vi "WPI_DigitalOutputGetPWM.vi"(8 "error in (no error)":errorcluster, 11 "DigitalOutputDevRef":T1={"DIO Channel"=enum."DIO 1", "DevStatus"={"status"=FALSE, "code"=0, "source"=""}}) -> (0 "error out":errorcluster, 2 "PWM Duty Cycle":sgl, 3 "DigitalOutputDevRef":T1={"DIO Channel"=enum."DIO 1", "DevStatus"={"status"=FALSE, "code"=0, "source"=""}})   [LabVIEW 2017]
doc: "Generates a PWM signal on a Digital Output channel.\n\nThe resolution of the duty cycle is 8-bit for low frequencies (1kHz or less) but is reduced the higher the frequency of the PWM signal is.\n\nThis software is licensed. Open the labview\\readme\\WPI Robotics Library Open Source License.txt file for more information."
uses:
  <vilib>/Rock Robotics/WPI/DigitalOutput/WPI_DigitalOutputDevRef.ctl
  <vilib>/Rock Robotics/SystemInterfaces/DIO/FPGA_DIOChannel.ctl
  <vilib>/Rock Robotics/WPI/DigitalModule/WPI_DigitalModuleDIOCacheOp.ctl
  <vilib>/Rock Robotics/SystemInterfaces/System/FPGA_SystemGet.vi
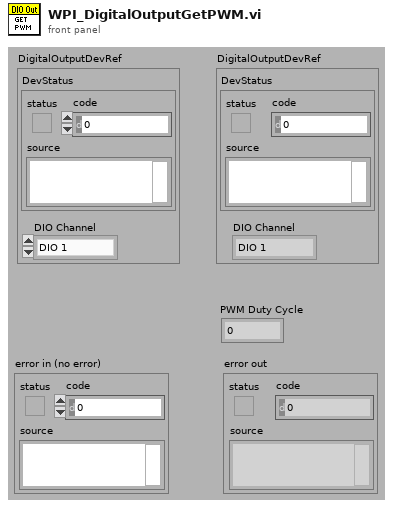
[diagram p1: front panel]
types:
  T1 = typedef "WPI_DigitalOutputDevRef.ctl" = cluster{"DIO Channel":T2, "DevStatus":errorcluster}
  T2 = typedef "FPGA_DIOChannel.ctl" = enum8{"DIO 0", "DIO 1", "DIO 2", "DIO 3", "DIO 4", "DIO 5", "DIO 6", "DIO 7", "DIO 8", "DIO 9", "DIO MXP 0", "DIO MXP 1", "DIO MXP 2", "DIO MXP 3", "DIO MXP 4", "DIO MXP 5", "DIO MXP 6", "DIO MXP 7", "DIO MXP 8", "DIO MXP 9", "DIO MXP 10", "DIO MXP 11", "DIO MXP 12", "DIO MXP 13", "DIO MXP 14", "DIO MXP 15", "SPI Port CS1", "SPI Port CS2", "SPI Port CS3", "SPI Port MISO", "SPI Port MOSI", "Invalid"}
  T3 = typedef "WPI_DigitalModuleDIOCacheOp.ctl" = enum16{"Acquire", "Release", "Status"}
  T4 = typedef "WPI_DigitalOutputPWMRef.ctl" = enum16{"DO PWM 0", "DO PWM 1", "DO PWM 2", "DO PWM 3", "DO PWM 4", "DO PWM 5", "Invalid"}
  T5 = typedef "FPGA_DIODevRef.ctl" = cluster{"DevStatus":errorcluster}
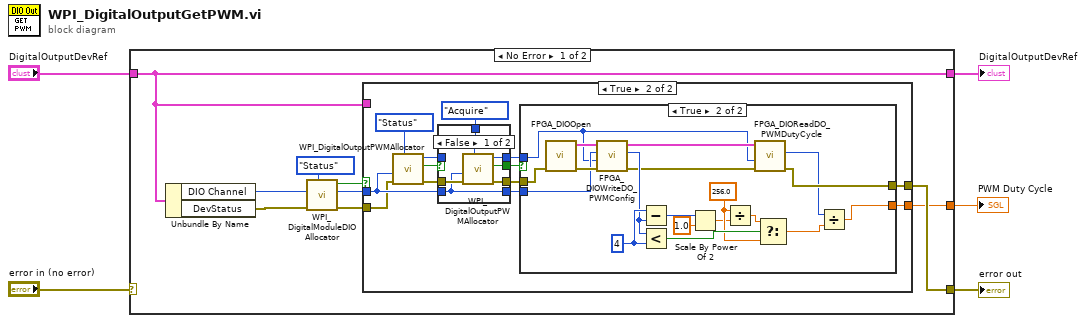
[diagram p0: block diagram]
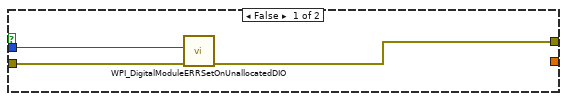
[diagram p2: hidden frame]
diagram:
  n1 = case shown="No Error" "error in (no error)" {
    selector: "error in (no error)" -> [_ w62]
    tunnel: "DigitalOutputDevRef" -> [w7 w61]
    tunnel: [w7 w61] -> w4
    tunnel: [w8 w62] -> w2
    tunnel: [w6 _] -> w1
    frame No Error {
      n2 = Unbundle By Name(w7) -> ("DIO Channel"=w13:T2, "DevStatus"=w12:errorcluster)
      n3 = call <vilib>:"WPI_DigitalModuleDIOAllocator.vi"("AllocatedDIOMutex"=WPI_DigitalModuleDIOCacheOp."Status", "error in (no error)"=w12, "DIOChannel"=w13) -> ("error out"=w9:errorcluster, "Allocated DIOChannel"=w11:T2, "AllocatedDIO"=w10:bool)  [unwired: 1 in, 5 out]
      n4 = case shown="True" w10 {
        tunnel: [w16 w19] -> w8
        tunnel: w11 -> [w15 w26]
        tunnel: w7 -> [_ _]
        tunnel: w9 -> [w17 w25]
        tunnel: [_ w18] -> w6
        frame False {
          n5 = call <vilib>:"WPI_DigitalModuleERRSetOnUnallocatedDIO.vi"("error in (no error)"=w17, "DIOChannel"=w15) -> ("error out"=w16:errorcluster)  [unwired: 9 in]
        }
        frame True {
          n6 = call <vilib>:"WPI_DigitalOutputPWMAllocator.vi"("Operation"=WPI_DigitalModuleDIOCacheOp."Status", "error in (no error)"=w25, "DIO Channel"=w26) -> ("error out"=w24:errorcluster, "Allocated"=w29:bool, "PWM Allocated"=w28:T4)  [unwired: 2 in, 4 out]
          n7 = case shown="False" w29 {
            selector: w29 -> [_ w58]
            tunnel: w28 -> [_ w60]
            tunnel: [w56 w60] -> w22
            tunnel: WPI_DigitalModuleDIOCacheOp."Acquire" ("Operation") -> [w55 _]
            tunnel: w26 -> [w51 w57]
            tunnel: w24 -> [w54 w59]
            tunnel: [w53 w59] -> w20
            tunnel: [w52 w58] -> w23
            tunnel: [w51 w57] -> w21
            frame False {
              n8 = call <vilib>:"WPI_DigitalOutputPWMAllocator.vi"("Operation"=w55, "error in (no error)"=w54, "DIO Channel"=w51) -> ("error out"=w53:errorcluster, "Allocated"=w52:bool, "PWM Allocated"=w56:T4)  [unwired: 2 in, 4 out]
            }
            frame True {
            }
          }
          n9 = case shown="True" w23 {
            tunnel: w22 -> [_ w36]
            tunnel: w21 -> [_ w47]
            tunnel: w20 -> [w31 w49]
            tunnel: [w31 w33] -> w19
            tunnel: [_ w34] -> w18
            frame False {
            }
            frame True {
              w45 = u8 4 ("y")
              w43 = 256.0 ("y")
              n10 = call <vilib>:"FPGA_DIOOpen.vi"("error in (no error)"=w49) -> ("error out"=w48:errorcluster, "DIODeviceRef"=w50:T5)  [unwired: 1 in, 8 out]
              n11 = call <vilib>:"FPGA_DIOWriteDO_PWMConfig.vi"("error in (no error)"=w48, "DO_PWM Index"=w36, "DO_PWMOutputSelect"=w47, "DIODeviceRef"=w50) -> ("error out"=w37:errorcluster, "DO_PWMPeriodPower Out"=w44:u16, "DIODeviceRef"=w38:T5)  [unwired: 1 in, 4 out]
              n12 = Subtract(x=w45, y=w44) -> (x-y=w40:u16)
              n13 = Less?(x=w44, y=w45) -> (x < y?=w46:bool)
              n14 = Scale By Power Of 2(n=w40, x=1.0) -> (x*2^n=w39:dbl)
              n15 = Divide(x=w43, y=w39) -> (x/y=w42:dbl)
              n16 = call <vilib>:"FPGA_DIOReadDO_PWMDutyCycle.vi"("error in (no error)"=w37, "DO_PWM Index"=w36, "DIODeviceRef"=w38) -> ("error out"=w33:errorcluster, "DO_PWMDutyCycle"=w32:u8)  [unwired: 6 in, 1 out]
              n17 = Select(t=w42, s=w46, f=w43) -> (s? t:f=w35:dbl)
              n18 = Divide(x=w32, y=w35) -> (x/y=w34:dbl)
            }
          }
        }
      }
    }
    frame Error {
    }
  }
  "DigitalOutputDevRef" <- w4
  "error out" <- w2
  "PWM Duty Cycle" <- w1
